vi "Launch Server Client Loop.vi"(3 "Event Logging":refnum<class "EventLoggingService.lvclass">, 4 "Local Version":string, 5 "TCPMessageAPI":refnum<class "TCPMessageAPI.lvclass">, 6 "Client Action Q":refnum<queue>, 7 "Fwd Queue":refnum<queue>, 8 "TCP Client":refnum<k5>, 9 "Remote Port":u16, 10 "Remote Address":string, 11 "Conn Handlers":refnum<queue>) -> (0 "error out":errorcluster)   [LabVIEW 2020, in "Vecto.lvlib" / "TCPMessaging.lvclass"]
uses:
  TCPMessaging.lvclass
  TX Payload.ctl
  Client Action Data.ctl
  Client Action.ctl
  Client Info.ctl
  proto/TcpClientHello/Data.ctl
  TCPMessageService/TCPMessageAPI.lvclass
  TCPConnectionHandler/TCPConnectionHandler.lvclass
  Server Client Loop.vi
  TCPMessaging.lvclass/TCPMessaging.ctl
  proto/TcpClientHello/TcpClientHello.lvlib
  VectoConfig/VectoConfig.lvlib
  Vecto.lvlib
  EventLoggingService/EventLoggingService.lvclass
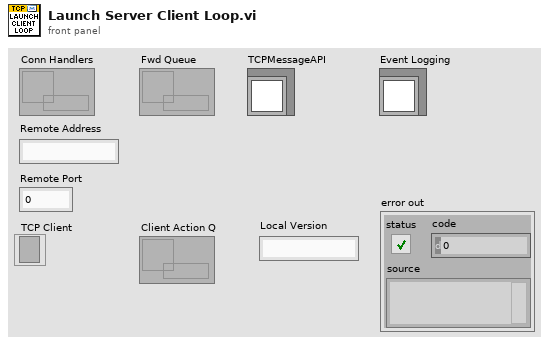
[diagram p1: front panel]
types:
  T1 = typedef "Vecto.lvlib/TCPMessaging.lvclass/Client Action.ctl" = enum16{"Connect", "Ready", "Disconnect"}
  T2 = typedef "Vecto.lvlib/TCPMessaging.lvclass/Client Action Data.ctl" = cluster{"Client Action":T1, "Client Info":T3, "TCP":refnum<k5>, "TX Q":refnum<queue>}
  T3 = typedef "VectoConfig.lvlib/Client Info.ctl" = cluster{"TcpClientHello":T4, "Remote Address":string, "Remote Port":u16}
  T4 = typedef "TcpClientHello.lvlib/Data.ctl" = cluster{"node_id":u32, "system":string, "cluster":string, "node_name":string, "app_version":string, "config_version":string}
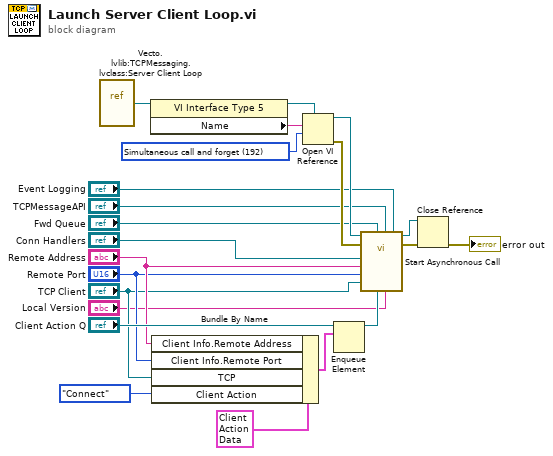
[diagram p0: block diagram]
diagram:
  w17 = 192 items=["Record modifications"=1, "Open templates for editing"=2, "Prompt user to save"=4, "Prepare for reentrant run"=8, "Prompt to find missing subVIs"=16, "Hide loading dialog box"=32, "Enable simultaneous calls"=64, "Prepare to call and forget"=128, "Simultaneous call and forget"=192, "Prepare to call and collect"=256, "Simultaneous call and collect"=320]
  n1 = vi-ref "Vecto.lvlib:TCPMessaging.lvclass:Server Client Loop.vi"() -> (w15:refnum<vi>)
  n2 = property class="VI Interface Type 5"(reference=w15) -> (reference out=w18:refnum<vi>, "Name"=w16:string)  [unwired: 1 in, 1 out]
  n3 = Bundle By Name(cluster=T2 {"Client Action"=enum."Disconnect", "Client Info"={"TcpClientHello"={"node_id"=0, "system"="", "cluster"="", "node_name"="", "app_version"="", "config_version"=""}, "Remote Address"="", "Remote Port"=0}, "TCP"=refnum, "TX Q"=refnum} ("element"), "Client Info.Remote Address"="Remote Address", "Client Info.Remote Port"="Remote Port", "TCP"="TCP Client", "Client Action"=Client_Action."Connect") -> (w9:T2)
  n4 = Open VI Reference(type specifier VI Refnum (for type only)=w18, vi path=w16, options=w17) -> (vi reference=w20:refnum<vi>, error out=w19:errorcluster)  [unwired: 3 in]
  n5 = Enqueue Element(queue="Client Action Q", element=w9) -> (queue out=w11:refnum<queue>)  [unwired: 2 in, 2 out]
  n6 = call-by-ref "Start Asynchronous Call"(reference=w20, error in=w19, "EventLogging"="Event Logging", "Local Version"="Local Version", "TCPMessageAPI"="TCPMessageAPI", "Client Action Q"=w11, "Fwd Queue"="Fwd Queue", "TCP Client"="TCP Client", "Remote Port"="Remote Port", "Remote Address"="Remote Address", "Conn Handlers"="Conn Handlers") -> (reference out=w22:refnum<vi>, error out=w21:errorcluster)  [unwired: 3 in]
  n7 = Close Reference(reference=w22, error in (no error)=w21) -> (error out=→"error out":errorcluster)
